vi "Test App Remove Deeply Nested Process by Qualified Name from Middle.vi"(8 "error in (no error)":errorcluster, 11 "Application Test in":refnum<class "Application Test.lvclass">) -> (0 "error out":errorcluster, 3 "Application Test out":refnum<class "Application Test.lvclass">)   [LabVIEW 2020, in "Application Test.lvclass"]
uses:
  Application Test.lvclass
  Framework/Process/Process.lvclass
  Framework/Application/Application.lvclass
  <vilib>/Asteme/LUnit/Test Case.lvclass
  C:/Users/anton/Documents/GitHub/Triarc-Framework/source/Framework/Process/Process.lvclass
  C:/Users/anton/Documents/GitHub/Triarc-Framework/source/Framework/Base/Base.lvclass
  C:/Users/anton/Documents/GitHub/Triarc-Framework/source/Framework/Error Handler Interface/Error Handler Interface.lvclass
  C:/Users/anton/Documents/GitHub/Triarc-Framework/source/Framework/Logging/Logging.lvclass
  C:/Users/anton/Documents/GitHub/Triarc-Framework/source/Framework/Application/Application.lvclass
  C:/Users/anton/Documents/GitHub/Triarc-Framework/source/Framework/Async Handler/Async Handler.lvclass
  C:/Users/anton/Documents/GitHub/Triarc-Framework/source/Framework Test/Process Test/Process Test.lvclass
  C:/Users/anton/Documents/GitHub/Triarc-Framework/source/Framework Test/Base Class Test/Base Test.lvclass
  C:/Program Files (x86)/National Instruments/LabVIEW 2020/vi.lib/Asteme/LUnit/Test Case.lvclass
  C:/Users/anton/Documents/GitHub/Triarc-Framework/source/Framework Test/Application Test/Application Test.lvclass
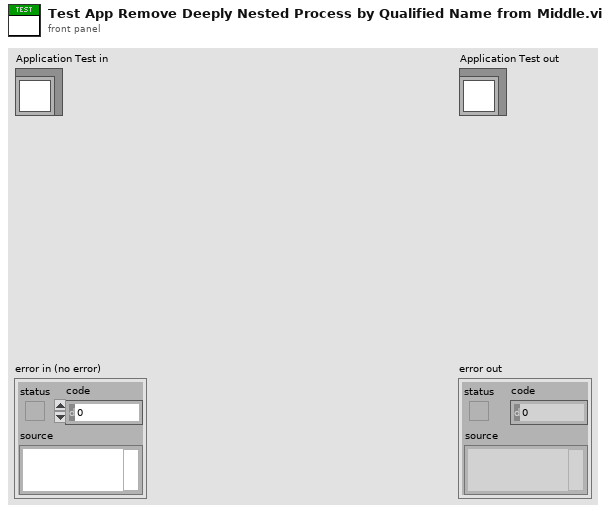
[diagram p1: front panel]
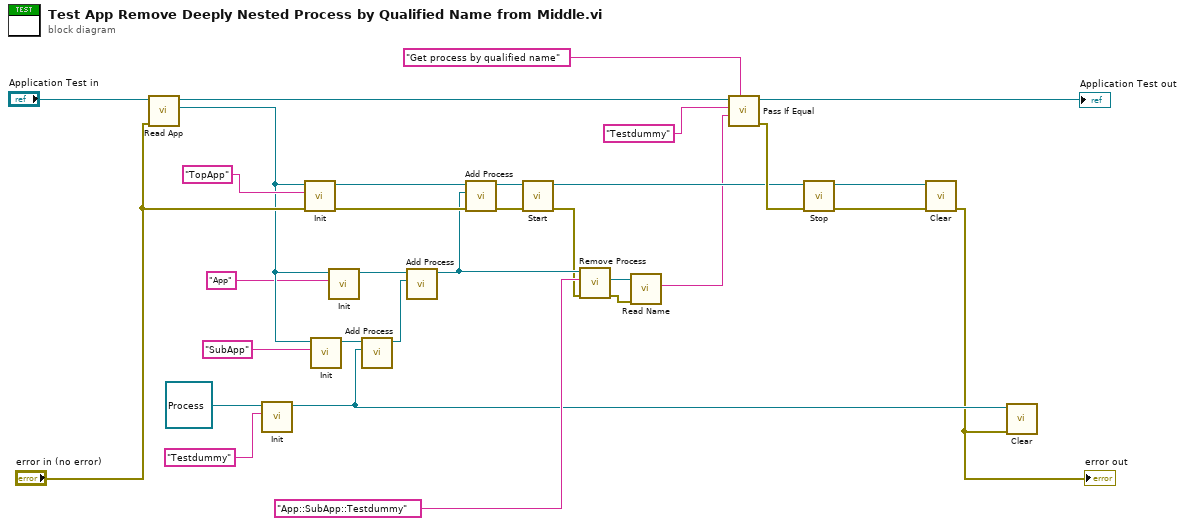
[diagram p0: block diagram]
diagram:
  n1 = call "Read App.vi"("error in (no error)"="error in (no error)", "Application Test In"="Application Test in") -> ("App out"=w16:refnum<class "Application.lvclass">, "Application Test Out"=w31:refnum<class "Application Test.lvclass">)  [unwired: 7 in, 1 out]
  n2 = call-dynamic "Init.vi"("Name"="Testdummy", "Process In"=refnum<class "Process.lvclass"> refnum ("Process.lvclass")) -> ("Process Out"=w6:refnum<class "Process.lvclass">)  [unwired: 8 in, 1 out]
  n3 = call-dynamic "Init.vi"("error in (no error)"="error in (no error)", "Name"="TopApp", "Process In"=w16) -> ("error out"=w29:errorcluster, "Process Out"=w30:refnum<class "Application.lvclass">)  [unwired: 7 in]
  n4 = call-dynamic "Init.vi"("Name"="SubApp", "Process In"=w16) -> ("Process Out"=w17:refnum<class "Application.lvclass">)  [unwired: 8 in, 1 out]
  n5 = call-dynamic "Init.vi"("Name"="App", "Process In"=w16) -> ("Process Out"=w15:refnum<class "Application.lvclass">)  [unwired: 8 in, 1 out]
  n6 = call "Add Process.vi"("Process"=w6, "Rig In"=w17) -> ("Rig Out"=w14:refnum<class "Application.lvclass">)  [unwired: 8 in, 1 out]
  n7 = call "Add Process.vi"("Process"=w14, "Rig In"=w15) -> ("Rig Out"=w12:refnum<class "Application.lvclass">)  [unwired: 8 in, 1 out]
  n8 = call "Add Process.vi"("error in (no error)"=w29, "Process"=w12, "Rig In"=w30) -> ("error out"=w11:errorcluster, "Rig Out"=w8:refnum<class "Application.lvclass">)  [unwired: 7 in]
  n9 = call "Start.vi"("error in (no error)"=w11, "Process In"=w8) -> ("error out"=w9:errorcluster, "Process Out"=w7:refnum<class "Application.lvclass">)  [unwired: 7 in, 1 out]
  n10 = call "Remove Process.vi"("error in (no error)"=w9, "Process Name"="App::SubApp::Testdummy" ("Name"), "Rig In"=w12) -> ("error out"=w1:errorcluster, "App Process"=w3:refnum<class "Process.lvclass">)  [unwired: 6 in, 1 out]
  n11 = call "Read Name.vi"("error in (no error)"=w1, "Process In"=w3) -> ("Qualified Name"=w2:string)  [unwired: 6 in, 3 out]
  n12 = call <vilib>:"Pass If Equal.vi"("Description"="Get process by qualified name", "Actual"=w2, "Expected"="Testdummy" ("Name"), "Test Case In"=w31) -> ("error out"=w25:errorcluster, "Test Case Out"=→"Application Test out":refnum<class "Application Test.lvclass">)  [unwired: 6 in]
  n13 = call "Stop.vi"("error in (no error)"=w25, "Process In"=w7) -> ("error out"=w23:errorcluster, "Process Out"=w28:refnum<class "Application.lvclass">)  [unwired: 7 in, 1 out]
  n14 = call-dynamic "Clear.vi"("error in (no error)"=w23, "Application In"=w28) -> ("error out"=w5:errorcluster)  [unwired: 9 in]
  "error out" <- w5
  n15 = call-dynamic "Clear.vi"("error in (no error)"=w5, "Process In"=w6) -> ()  [unwired: 9 in, 1 out]
